vi "Get App Info.vi"(8 "error in":errorcluster caption="Error In", 10 "Build Spec Name":string, 11 "Project Path":path) -> (0 "error out":errorcluster caption="Error Out", 1 "Description":string, 2 "Version":string, 3 "Vendor":string, 4 "Architecture":string)   [LabVIEW 2016]
doc: "Open the VI reference pointed by the VI Name input. This function does not require a path as input but requires that the VI is present in the same project as the calling VI."
panel:
  out "Tag:Get Names":string[](array[string])
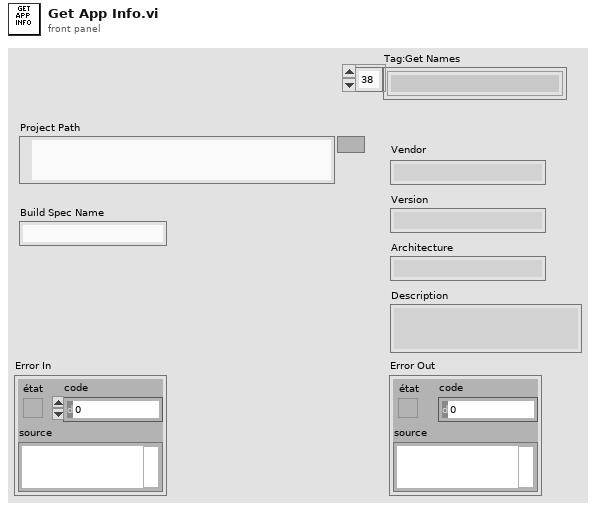
[diagram p1: front panel]
types:
  T1 = enum32{"invalid CPU target", "Motorola 68K", "PowerPC", "Intel x86", "SPARC", "PA-RISC", "MIPS", "Alpha", "ARM", "AMD/Intel x64"}
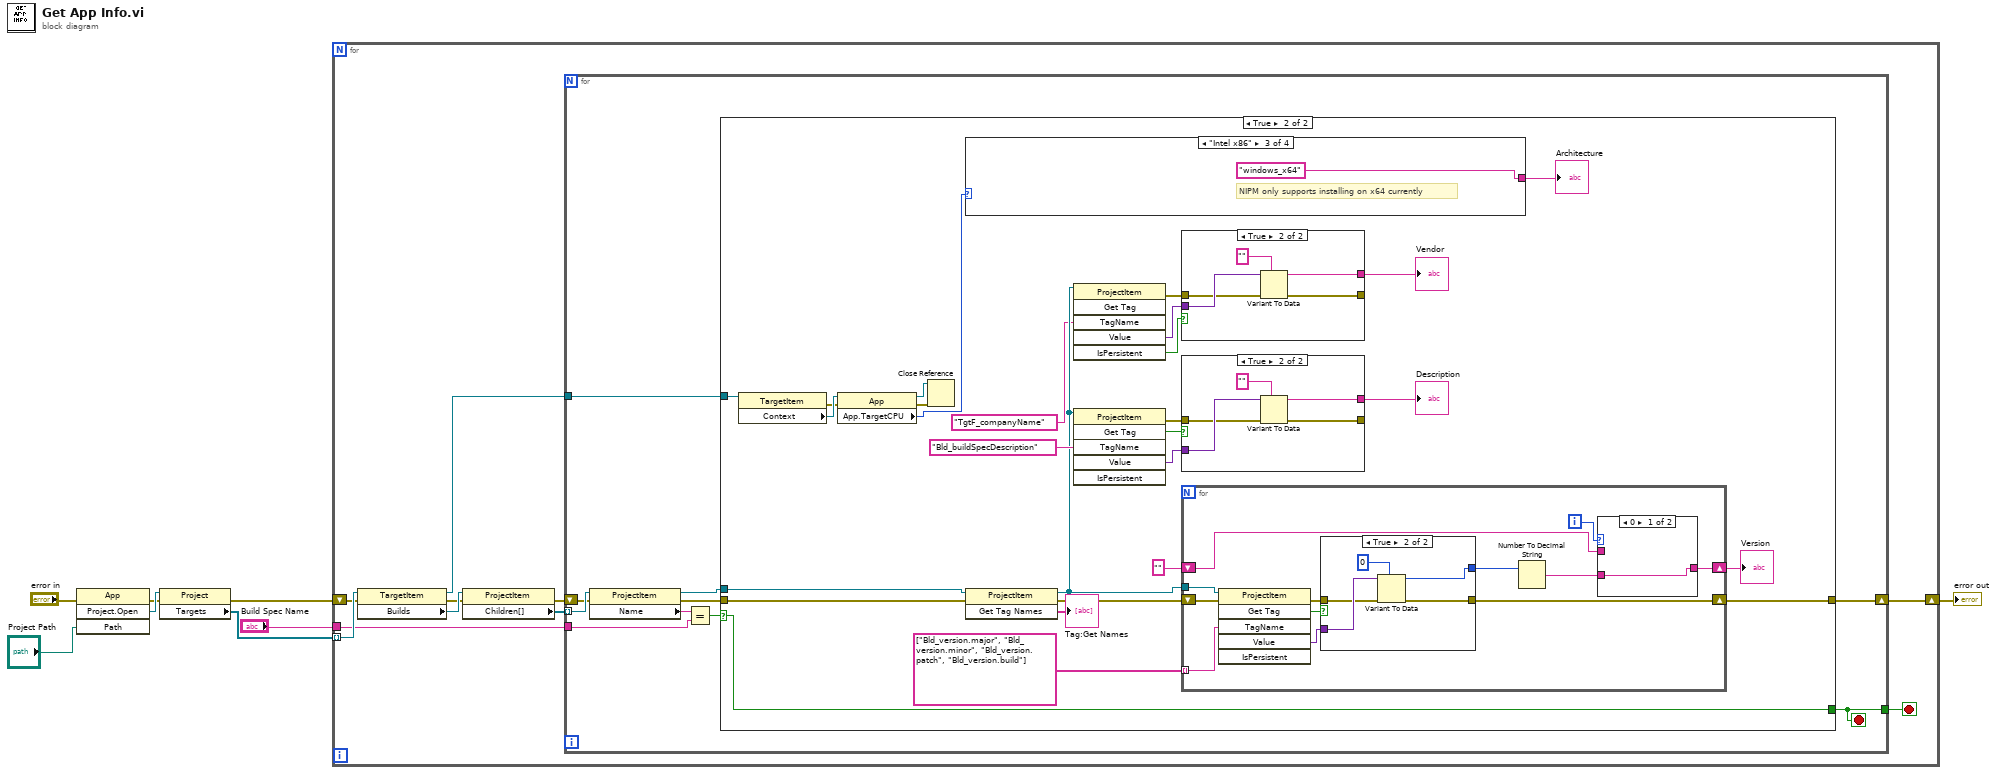
[diagram p0: block diagram]
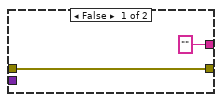
[diagram p3: hidden frame]
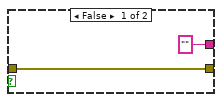
[diagram p4: hidden frame]
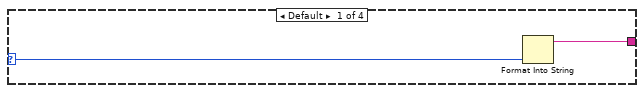
[diagram p5: hidden frame]
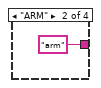
[diagram p6: hidden frame]
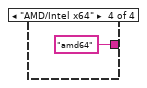
[diagram p7: hidden frame]
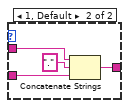
[diagram p8: hidden frame]
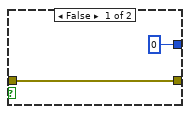
[diagram p9: hidden frame]
diagram:
  n1 = invoke class="App" method="Project.Open"(error in="error in", "Path"="Project Path") -> (error out=w5:errorcluster, "Project:Open"=w6:refnum<vi>)  [unwired: 2 in, 2 out]
  n2 = property class="Project"(reference=w6, error in=w5) -> (error out=w3:errorcluster, "Targets"=w8:refnum<vi>[])  [unwired: 1 out]
  n3 = for {
    tunnel: w8 -> [w18] mode=indexing
    tunnel: "Build Spec Name" -> [w15]
    shift-right: [w10] -> w2
    shift-left: w3 -> [w11]
    stop <- w13 stop-if-true
    n4 = property class="TargetItem"(reference=w18, error in=w11) -> (reference out=w9:refnum<vi>, error out=w14:errorcluster, "Builds"=w17:refnum<vi>)
    n5 = property class="ProjectItem"(reference=w17, error in=w14) -> (error out=w12:errorcluster, "Children[]"=w16:refnum<vi>[])  [unwired: 1 out]
    n6 = for {
      tunnel: w16 -> [w26] mode=indexing
      tunnel: w15 -> [w27]
      tunnel: [w24] -> w13
      shift-right: [w20] -> w10
      shift-left: w12 -> [w23]
      tunnel: w9 -> [w19]
      stop <- w24 stop-if-true
      n7 = property class="ProjectItem"(reference=w26, error in=w23) -> (reference out=w21:refnum<vi>, error out=w22:errorcluster, "Name"=w28:string)
      n8 = Equal?(x=w28, y=w27) -> (x = y?=w25:bool)
      n9 = case shown="True" w25 {
        selector: w25 -> [_ w55]
        tunnel: w21 -> [_ w56]
        tunnel: [_ w55] -> w24
        tunnel: w22 -> [w29 w52]
        tunnel: [w29 w50] -> w20
        tunnel: w19 -> [_ w45]
        frame False {
        }
        frame True {
          n10 = property class="TargetItem"(reference=w45) -> (error out=w47:errorcluster, "Context"=w49:refnum<vi>)  [unwired: 1 in, 1 out]
          n11 = property class="App"(reference=w49, error in=w47) -> (reference out=w44:refnum<vi>, error out=w48:errorcluster, "App.TargetCPU"=w46:T1)
          n12 = Close Reference(reference=w44, error in (no error)=w48) -> ()  [unwired: 1 out]
          n13 = case shown="\"Intel x86\"" w46 {
            selector: w46 -> [w72 _ _ _]
            tunnel: [w71 "arm" "windows_x64" "amd64"] -> w43
            frame Default {
              n14 = Format Into String(w72) -> (resulting string=w71:string)  [unwired: 3 in, 1 out]
            }
            frame "ARM" {
            }
            frame "Intel x86" {
              # "NIPM only supports installing on x64 currently"
            }
            frame "AMD/Intel x64" {
            }
          }
          "Architecture" <- w43
          n15 = invoke class="ProjectItem" method="Get Tag Names"(reference=w56, error in=w52) -> (reference out=w36:refnum<vi>, error out=w51:errorcluster, "Get Tag Names"=→"Tag:Get Names":string[])  [unwired: 1 in]
          n16 = invoke class="ProjectItem" method="Get Tag"(reference=w36, "TagName"="TgtF_companyName" ("Tag Name")) -> (error out=w34:errorcluster, "Value"=w33:variant, "IsPersistent"=w31:bool)  [unwired: 4 in, 3 out]
          n17 = invoke class="ProjectItem" method="Get Tag"(reference=w36, "TagName"="Bld_buildSpecDescription") -> (error out=w38:errorcluster, "GetTag"=w40:bool, "Value"=w39:variant)  [unwired: 4 in, 3 out]
          n18 = case shown="True" w31 {
            tunnel: [w57 w63] -> _
            tunnel: w33 -> [_ w61]
            tunnel: ["" w60] -> w32
            tunnel: w34 -> [w57 w59]
            frame False {
            }
            frame True {
              n19 = Variant To Data(error in=w59, type="", Variant=w61) -> (data=w60:string, error out=w63:errorcluster)
            }
          }
          "Vendor" <- w32
          n20 = case shown="True" w40 {
            tunnel: [w64 w70] -> _
            tunnel: w39 -> [_ w68]
            tunnel: ["" w67] -> w37
            tunnel: w38 -> [w64 w66]
            frame False {
            }
            frame True {
              n21 = Variant To Data(error in=w66, type="", Variant=w68) -> (data=w67:string, error out=w70:errorcluster)
            }
          }
          "Description" <- w37
          n22 = for {
            tunnel: w36 -> [w86]
            tunnel: string[] ["Bld_version.major", "Bld_version.minor", "Bld_version.patch", "Bld_version.build"] -> [w85] mode=indexing
            shift-right: [w80] -> w42
            shift-left: "" -> [w81]
            shift-right: [w76] -> w50
            shift-left: w51 -> [w78]
            i -> [w79]
            n23 = invoke class="ProjectItem" method="Get Tag"(reference=w86, error in=w78, "TagName"=w85) -> (error out=w77:errorcluster, "GetTag"=w84:bool, "Value"=w87:variant)  [unwired: 3 in, 3 out]
            n24 = case shown="True" w84 {
              tunnel: w87 -> [_ w99]
              tunnel: [0 w97] -> w83
              tunnel: w77 -> [w93 w96]
              tunnel: [w93 w95] -> w76
              frame False {
              }
              frame True {
                n25 = Variant To Data(error in=w96, type=0, Variant=w99) -> (data=w97:i32, error out=w95:errorcluster)
              }
            }
            n26 = Number To Decimal String(number=w83) -> (decimal integer string=w82:string)  [unwired: 1 in]
            n27 = case shown="0" w79 {
              tunnel: w82 -> [w88 w92]
              tunnel: w81 -> [_ w90]
              tunnel: [w88 w91] -> w80
              frame 0 {
              }
              frame 1, Default {
                n28 = Concatenate Strings(w90, "." ("string"), w92) -> (w91:string)
              }
            }
          }
          "Version" <- w42
        }
      }
    }
  }
  "error out" <- w2
